vi "ReadMessage.vi"() -> ()   [LabVIEW 2014]
uses:
  Program Files (x86)/National Instruments/LabVIEW 2014/examples/Instrument IO/Serial/support/Serial - Settings.ctl
  <vilib>/Instr/_visa.llb/VISA Configure Serial Port (Instr).vi
panel:
  in  "VISA resource name":refnum<visa-resource-name>="COM1"
  in  "Serial Settings":T1={"baud rate"=9600, "data bits"=8, "parity"=enum."None", "stop bits"=10, "flow control"=0} {"flow control" items=["None"=0, "XON/XOFF"=1, "RTS/CTS"=2, "DTR/DSR"=4]; "stop bits" items=["1.0"=10, "1.5"=15, "2.0"=20]; "data bits" min=5 max=8 step=1; "baud rate" items=["75"=75, "110"=110, "134"=134, "150"=150, "300"=300, "600"=600, "1200"=1200, "1800"=1800, "2400"=2400, "4800"=4800, "7200"=7200, "9600"=9600, "14400"=14400, "19200"=19200, "28800"=28800, "38400"=38400, "56000"=56000, "57600"=57600, "115200"=115200, "128000"=128000, "230400"=230400]}
  out "Response":string
  in  "Read Count":u32=1000
  in  "Command":string="*IDN?"
  in  "Read":bool
  in  "Stop":bool
  in  "Write":bool
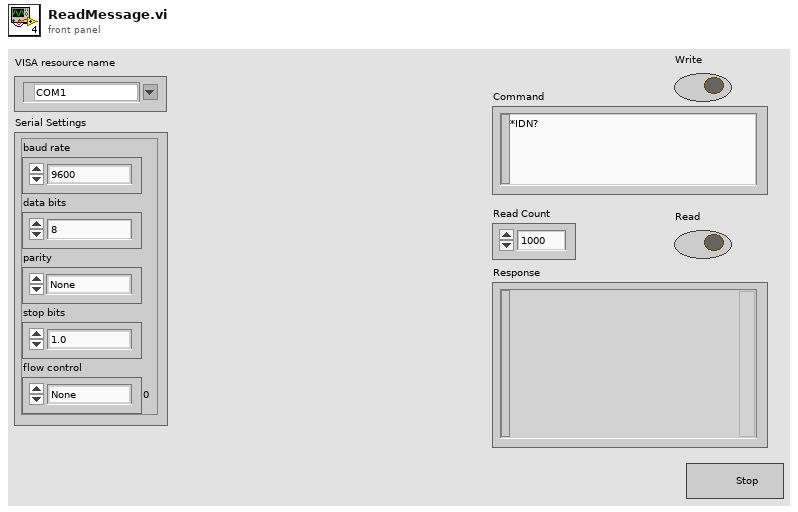
[diagram p1: front panel]
types:
  T1 = typedef "Serial - Settings.ctl" = cluster{"baud rate":u32, "data bits":u16, "parity":enum16{"None", "Odd", "Even", "Mark", "Space"}, "stop bits":u16, "flow control":u16}
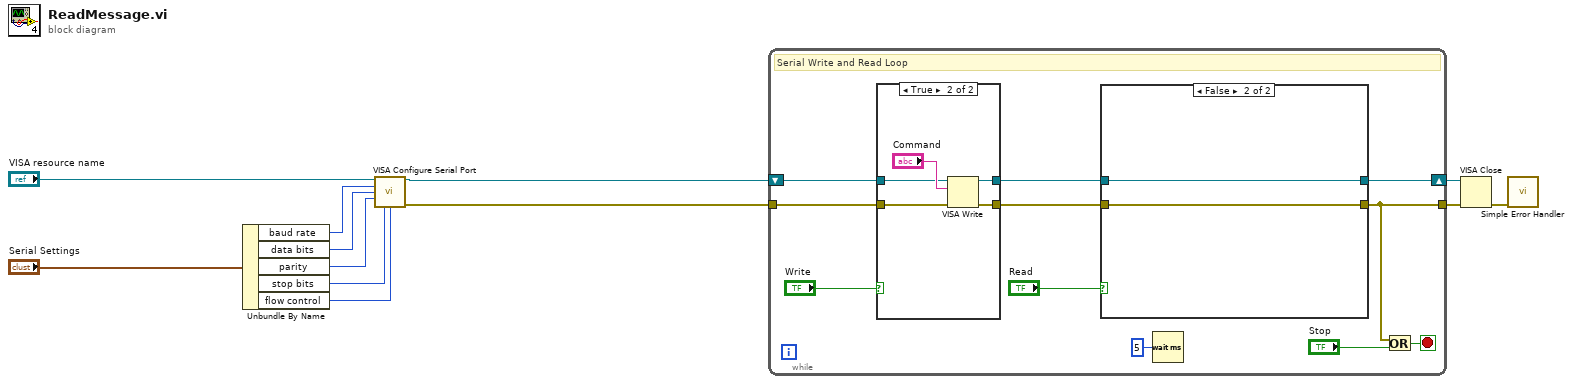
[diagram p0: block diagram]
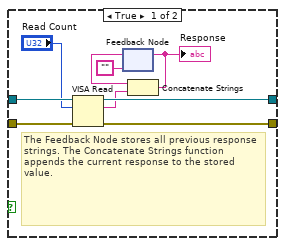
[diagram p3: hidden frame]
diagram:
  n1 = Unbundle By Name("Serial Settings") -> ("baud rate"=w8:u32, "data bits"=w9:u16, "parity"=w10:enum16{"None", "Odd", "Even", "Mark", "Space"}, "stop bits"=w11:u16, "flow control"=w3:u16)
  n2 = call-poly "VISA Configure Serial Port"("VISA resource name"="VISA resource name", "baud rate (9600)"=w8, "data bits (8)"=w9, "parity (0:none)"=w10, "stop bits (10: 1 bit)"=w11, "flow control (0:none)"=w3) -> ("VISA resource name out"=w2:refnum<visa-resource-name>, "error out"=w1:errorcluster)  [unwired: 4 in, 4 out]
  n3 = while {
    shift-right: [w23] -> w4
    shift-left: w2 -> [w22]
    tunnel: [w16] -> w5
    tunnel: w1 -> [w13]
    stop <- w17 stop-if-true
    # "Serial Write and Read Loop"
    n4 = case shown="True" "Write" {
      tunnel: w22 -> [w25 w29]
      tunnel: [w25 w28] -> w21
      tunnel: [w24 w27] -> w20
      tunnel: w13 -> [w24 w26]
      frame False {
      }
      frame True {
        n5 = VISA Write(VISA resource name=w29, write buffer="Command", error in (no error)=w26) -> (VISA resource name out=w28:refnum<visa-resource-name>, error out=w27:errorcluster)  [unwired: 1 out]
      }
    }
    n6 = case shown="False" "Read" {
      tunnel: [w37 w41] -> w23
      tunnel: w21 -> [w39 w41]
      tunnel: [w35 w40] -> w16
      tunnel: w20 -> [w38 w40]
      frame True {
        # "The Feedback Node stores all previous response strings. The Concatenate Strings function appends the current response to the stored value."
        n7 = VISA Read(VISA resource name=w39, byte count="Read Count", error in (no error)=w38) -> (VISA resource name out=w37:refnum<visa-resource-name>, read buffer=w34:string, error out=w35:errorcluster)  [unwired: 1 out]
        n8 = feedback #1("") -> (w33:string)
        n9 = Concatenate Strings(w33, w34) -> (w32:string)
        "Response" <- w32
        n10 = feedback-in #1(w32) -> ()
      }
      frame False {
      }
    }
    n11 = Wait (ms)(milliseconds to wait=u32 5) -> ()  [unwired: 1 out]
    n12 = Or(x=w16, y="Stop") -> (x .or. y?=w17:bool)
  }
  n13 = VISA Close(VISA resource name=w4, error in (no error)=w5) -> (error out=w6:errorcluster)
  n14 = call <vilib>:"Simple Error Handler.vi"("error in (no error)"=w6) -> ()  [unwired: 1 in, 8 out]
